vi "VerifyUploadDialog.vi"(0 "Enable":bool=TRUE, 3 "Delay":dbl format="%.2f", 5 "error in (no error)":errorcluster) -> (17 "Delay":dbl format="%#g", 18 "Retry":bool, 19 "error out":errorcluster)   [LabVIEW 2010]
doc: "Displays a standard dialog box that prompts users to enter information, such as a user name and password.\n--------------------\n\nThis Express VI is configured as follows:\n\nMessage to Display to the User:Would you like to retry the upload? If there is a terminal window that displays timeout errors, press Control-C in the window and retry the upload with a shorter Delay value. If there is a window that states unable to access port, retry the upload with a longer Delay value. A good starting value for Delay is 1.0 seconds.\nThe inputs are: \nNumber: Delay"
panel:
  out "Message":string="Would you like to retry the upload?\n\nIf you see timout errors in a terminal window, press Control-C, and close the terminal.  Choose a shorter Delay value and retry the upload.\n\nIf you see an \"access denied\" or \"resource busy\" error, close the terminal window and choose a longer Delay value."
  in  "Cancel":bool
  in  "OK2":bool
  in  "OK1":bool
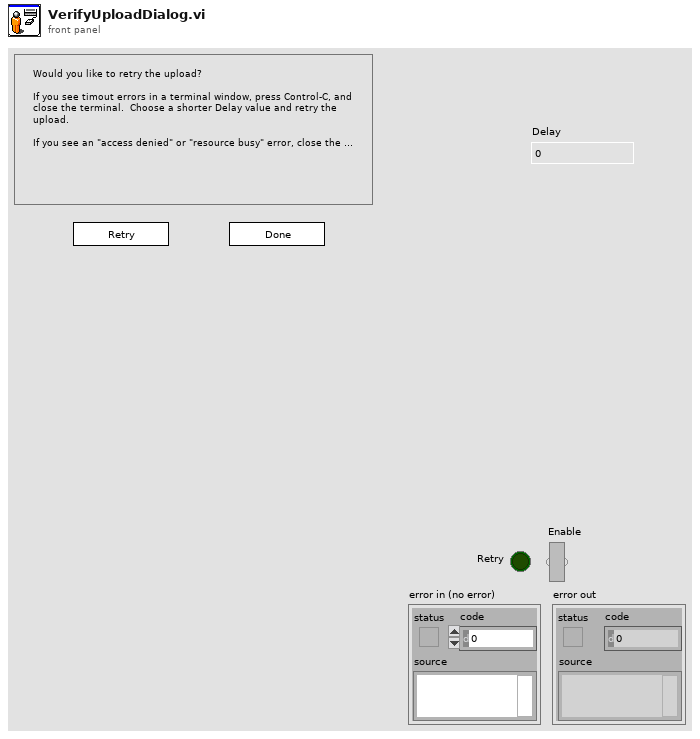
[diagram p1: front panel]
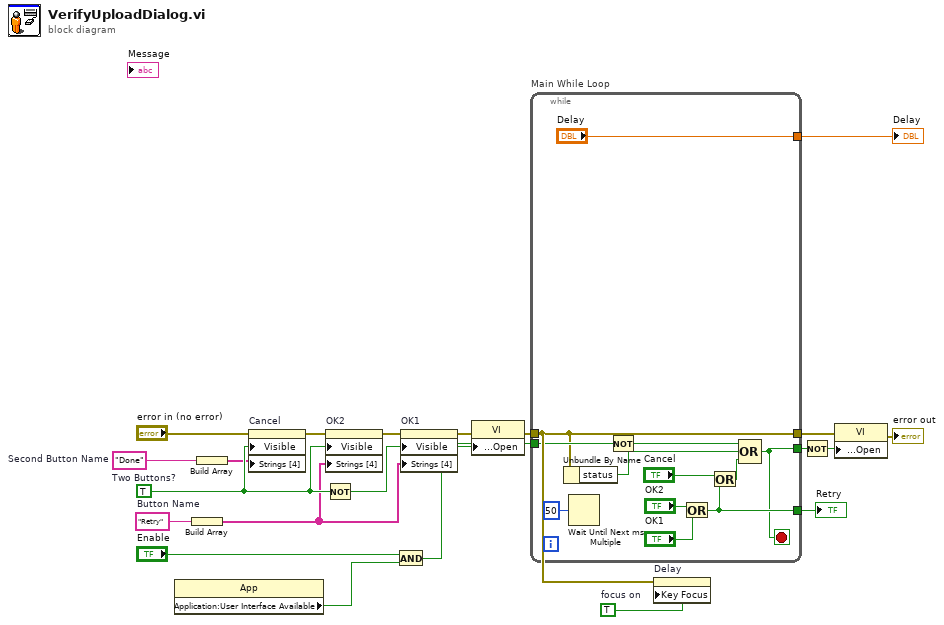
[diagram p0: block diagram]
diagram:
  w1 = TRUE  # focus on
  w13 = "Done"  # Second Button Name
  w11 = "Retry"  # Button Name
  w21 = TRUE  # Two Buttons?
  n1 = property class="App"() -> ("Application:User Interface Available"=w3:bool)  [unwired: 2 in, 2 out]
  n2 = Build Array(w11) -> (w12:string[])
  n3 = Build Array(w13) -> (w14:string[])
  n4 = property on="Cancel" class="Bool"(error in="error in (no error)", "Visible"=w21, "Strings [4]"=w14) -> (error out=w18:errorcluster)  [unwired: 1 in, 1 out]
  n5 = Not(x=w21) -> (.not. x?=w19:bool)
  n6 = property on="OK2" class="Bool"(error in=w18, "Visible"=w21, "Strings [4]"=w12) -> (error out=w17:errorcluster)  [unwired: 1 in, 1 out]
  n7 = And(x="Enable", y=w3) -> (x .and. y?=w4:bool)
  n8 = property on="OK1" class="Bool"(error in=w17, "Visible"=w19, "Strings [4]"=w12) -> (error out=w10:errorcluster)  [unwired: 1 in, 1 out]
  n9 = property class="VI"(error in=w10, "Front Panel Window:Open"=w4) -> (error out=w9:errorcluster)  [unwired: 1 in, 1 out]
  n10 = while "Main While Loop" {
    tunnel: [w30] -> w20
    tunnel: w4 -> [w28]
    tunnel: [w26] -> w15
    tunnel: w9 -> [w25]
    tunnel: [w25] -> w7
    tunnel: ["Delay"] -> w2
    stop <- w26 stop-if-true
    n11 = Unbundle By Name(w25) -> ("status"=w23:bool)
    n12 = Wait Until Next ms Multiple(millisecond multiple=u32 50) -> ()  [unwired: 1 out]
    n13 = Not(x=w28) -> (.not. x?=w27:bool)
    n14 = Or(x="OK2", y="OK1") -> (x .or. y?=w30:bool)
    n15 = Or(x="Cancel", y=w30) -> (x .or. y?=w24:bool)
    n16 = Compound Arithmetic op=OR(w27, w23, w24) -> (w26:bool)
  }
  "Retry" <- w20
  "Delay" <- w2
  n17 = property on="Delay" class="DigNum (strict)"(error in=w9, "Key Focus"=w1) -> ()  [unwired: 1 in, 2 out]
  n18 = Not(x=w15) -> (.not. x?=w16:bool)
  n19 = property class="VI"(error in=w7, "Front Panel Window:Open"=w16) -> (error out=→"error out":errorcluster)  [unwired: 1 in, 1 out]
